vi "Execute query.vi"(8 "error in (no error)":errorcluster, 10 "String":string="select GL_BREAKDOWN_IN_TIME\nfrom Plant_name.line_one_breakdown_history\nWhere month(GL_BREAKDOWN_IN_TIME) ='09' and  BREAKDOWN_MASTER_ID ='1'  and SHIFT_ID='1'  ", 11 "connection reference":T1) -> (0 "error out":errorcluster, 1 "Production Count":i32, 2 "Table":string[][](array[string]), 3 "connection reference 2":T1, 4 "ACTUAL  PLC PRODUCT CODE":i32, 5 "ACTUAL  PLC COUNT":i32)   [LabVIEW 2017]
uses:
  <vilib>/addons/database/Connection.llb/Conn ObjectReference.ctl
  <vilib>/addons/database/Connection.llb/Conn Execute.vi
  <vilib>/addons/database/Recordset.llb/Rec Fetch Recordset Data (R).vi
  <vilib>/addons/database/Recordset.llb/Rec Destroy - Connection.vi
  <userlib>/_OpenG.lib/array/array.llb/Search 1D Array (String)__ogtk.vi
  <userlib>/_OpenG.lib/array/array.llb/Delete Elements from 1D Array (String)__ogtk.vi
  <vilib>/addons/database/NI_Database_API.lvlib
panel:
  out "size(s) 2":i32[](array[numeric])
  in  "String 2":string="select GL_BREAKDOWN_IN_TIME\nfrom Plant_name.line_one_breakdown_history\nWhere month(GL_BREAKDOWN_IN_TIME) ='09' and  BREAKDOWN_MASTER_ID ='1'  and SHIFT_ID='1'  "
  in  "string":string="select PLAN_DATE\nfrom machine_and_shift_wise_daily_plan\nwhere month(PLAN_DATE)='%s' and year(PLAN_DATE)='%s'  and MACHINE_ID='%s'"
  # "Select* from  SERIAL_NUMBER"
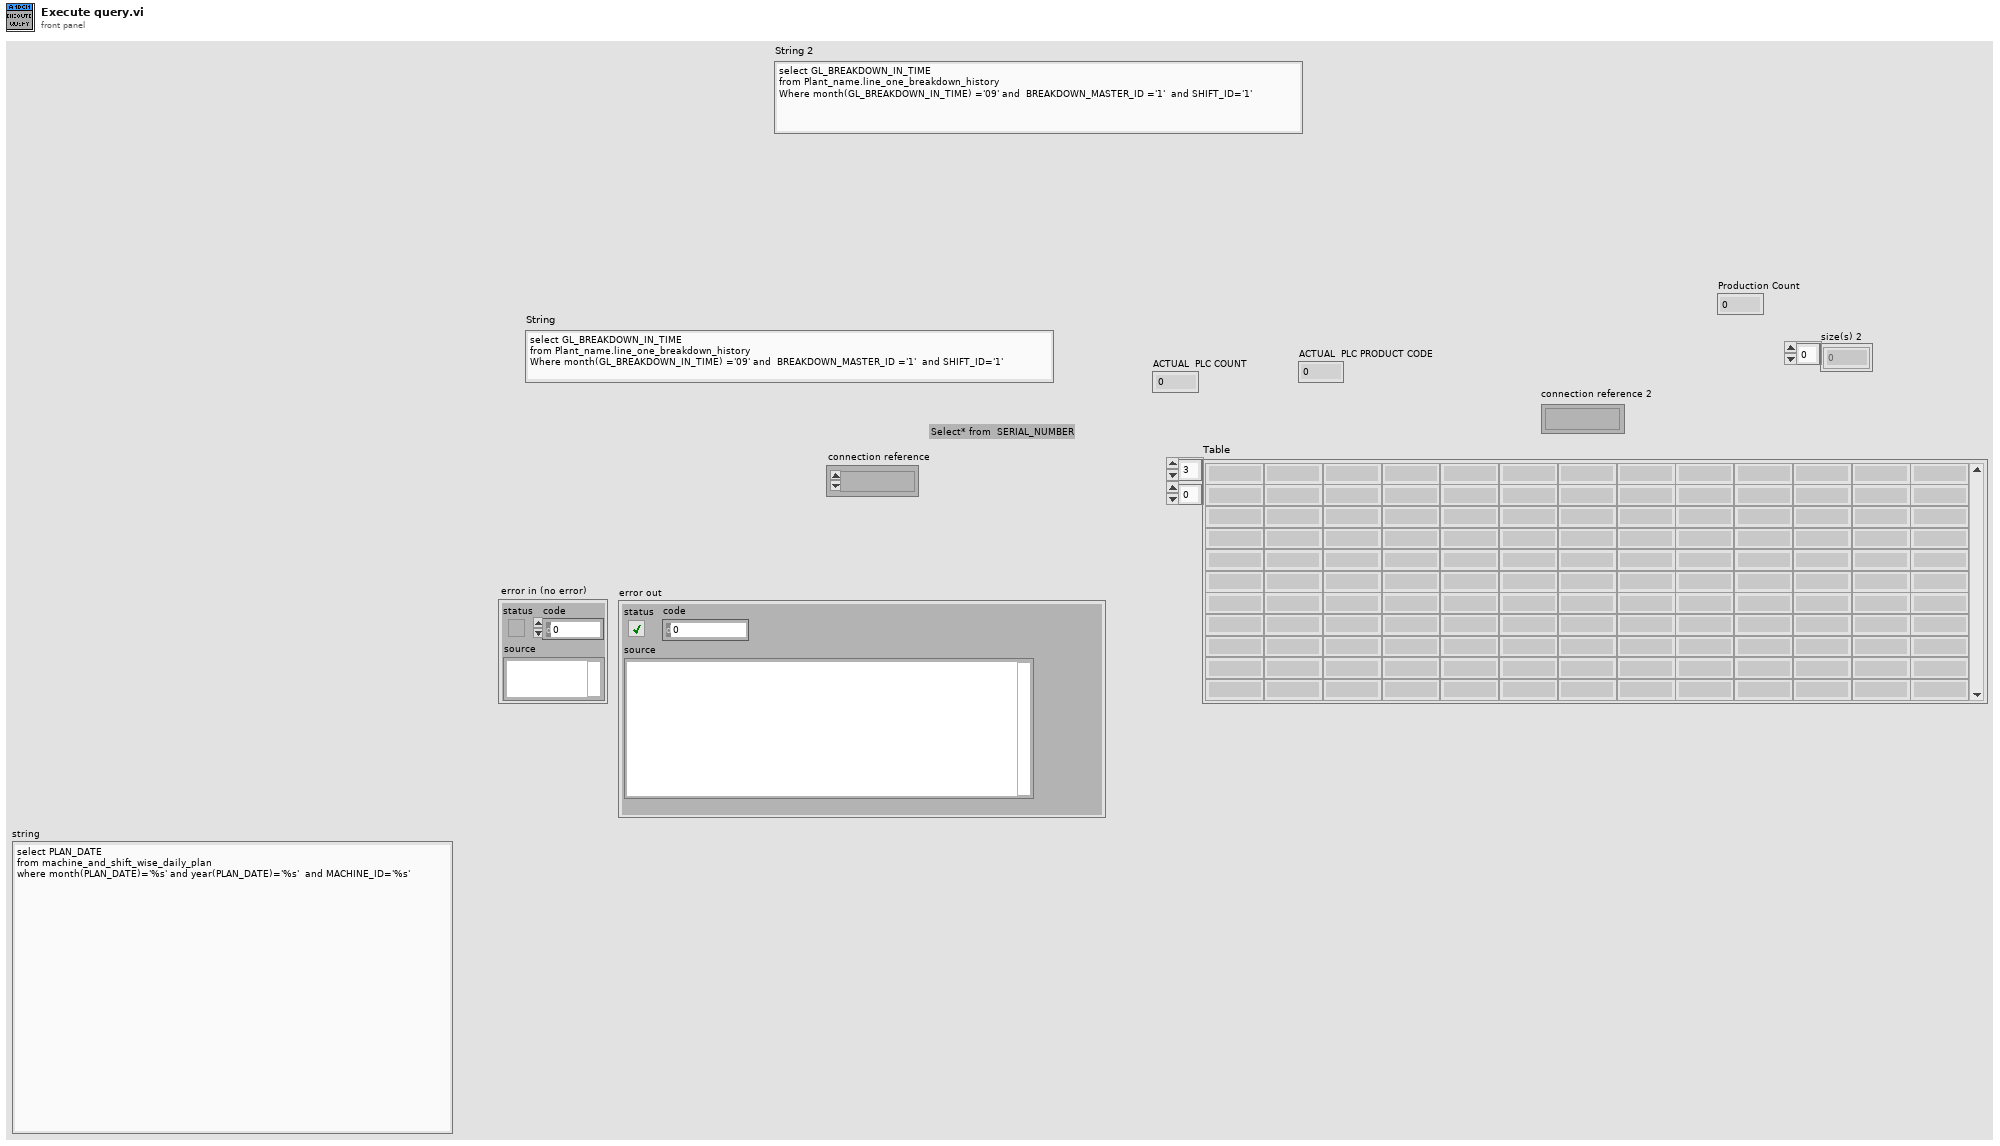
[diagram p1: front panel]
types:
  T1 = typedef "NI_Database_API.lvlib/Conn ObjectReference.ctl" = refnum<k1>
  T2 = typedef "NI_Database_API.lvlib/Rec ObjectReference.ctl" = refnum<k1>
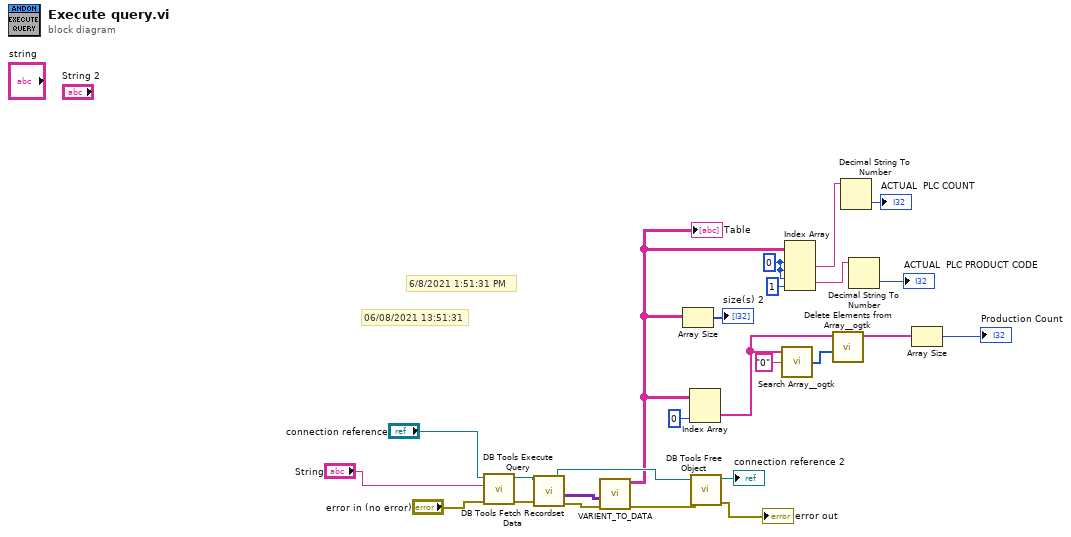
[diagram p0: block diagram]
diagram:
  w4 = 0 ("index (row)")
  # "06/08/2021 13:51:31"
  # "6/8/2021 1:51:31 PM"
  n1 = call-poly <vilib>:"DB Tools Execute Query.vi"("error in (no error)"="error in (no error)", "SQL query"="String", "connection reference"="connection reference") -> ("error out"=w25:errorcluster, "recordset reference"=w22:T2)  [unwired: 5 in]
  n2 = call-poly <vilib>:"DB Tools Fetch Recordset Data.vi"("error in (no error)"=w25, "recordset reference"=w22) -> ("error out"=w24:errorcluster, "recordset data"=w15:variant[][], "recordset reference out"=w21:T2)  [unwired: 3 in]
  n3 = call "VARIENT_TO_DATA.vi"("data"=w15, "error in (no error)"=w24) -> ("Table"=w7:string[][], "error out"=w20:errorcluster)  [unwired: 7 in]
  "Table" <- w7
  n4 = Array Size(array=w7) -> (size(s)=→"size(s) 2":i32[])
  n5 = Index Array(array=w7, index (col)=0 ("disabled index (col)")) -> (element=w11:string[])  [unwired: 1 in]
  n6 = call-poly <vilib>:"DB Tools Free Object.vi"("error in (no error)"=w20, "recordset reference"=w21) -> ("error out"=→"error out":errorcluster, "connection reference"=→"connection reference 2":T1)  [unwired: 8 in]
  n7 = call-poly <userlib>:"Search Array__ogtk.vi"("Array"=w11, "Element Data"="0") -> ("Indices of Elements"=w9:i32[])  [unwired: 7 in]
  n8 = Index Array(array=w7, index (row) #1=w4, index (col) #1=w4, index (row) #2=w4, index (col) #2=1 ("disabled index (col)")) -> (element #1=w6:string, element #2=w2:string)
  n9 = call-poly <userlib>:"Delete Elements from Array__ogtk.vi"("indices"=w9, "array"=w11) -> ("array w/ subset deleted"=w8:string[])  [unwired: 8 in, 1 out]
  n10 = Decimal String To Number(string=w6) -> (number=→"ACTUAL  PLC COUNT":i32)  [unwired: 2 in, 1 out]
  n11 = Decimal String To Number(string=w2) -> (number=→"ACTUAL  PLC PRODUCT CODE":i32)  [unwired: 2 in, 1 out]
  n12 = Array Size(array=w8) -> (size(s)=→"Production Count":i32)
